vi "Aurora Read Debug Signals (Dual Port).vi"(2 "Debug CLIP Resources":T2={"Hard Error"="Chevelle IO Socket\\uPort0_HardError", "Soft Error"="Chevelle IO Socket\\uPort0_SoftError", "Lane Up"="Chevelle IO Socket\\uPort0_LaneUp", "Channel Up"="Chevelle IO Socket\\uPort0_ChannelUp", "Sys Reset"="Chevelle IO Socket\\uPort0_sys_reset_out"}) -> (4 "Debug Info":T1)   [LabVIEW 2019]
doc: "Reads debug signals from the CLIP.\n\n<B>Input Parameters</B>\n\n<B>Debug CLIP Resources</B> specifies the CLIP Resources used for debug signals.\n\n<B>Debug CLIP Resources.Hard Error</B> specifies the CLIP Resource used to indicate a Hard Error.\n\n<B>Debug CLIP Resources.Soft Error</B> specifies the CLIP Resource used to indicate a Soft Error.\n\n<B>Debug CLIP Resources.Lane Up</B> specifies the CLIP Resource used to indicate whether the Lane is Up.\n\n<B>Debug CLIP Resources.Channel Up</B> specifies the CLIP Resource used to indicate whether the Channel is Up.\n\n<B>Debug CLIP Resources.Sys Reset</B> specifies the CLIP Resource used to indicate if the System is in Reset.\n\n<B>Output Parameters</B>\n\n<B>Debug Info</B> contains debug information read from the CLIP.\n\n<B>Debug Info.Hard Error</B> indicates whether a Hard Error has occurred.\n\n<B>Debug Info.Soft Error</B> indicates whether a Soft Error has occurred.\n\n<B>Debug Info.Lane Up</B> indicates whether the Lane is Up.\n\n<B>Debug Info.Channel Up</B> indicates whether the Channel is Up.\n\n<B>Debug Info.Sys Reset</B> indicates whether the System is in Reset."
uses:
  <vilib>/eio/EIONode/EIONode.xnode
  <vilib>/rvi/eio/common/nirviEmuTemplateMethod_errors.vi
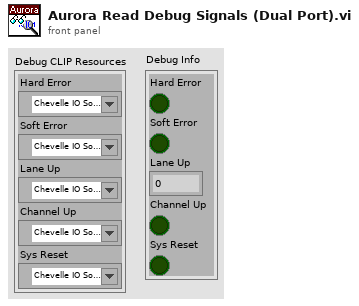
[diagram p1: front panel]
types:
  T1 = cluster{"Hard Error":bool, "Soft Error":bool, "Lane Up":fxp<+,8,8>, "Channel Up":bool, "Sys Reset":bool}
  T2 = cluster{"Hard Error":refnum<k21>, "Soft Error":refnum<k21>, "Lane Up":refnum<k21>, "Channel Up":refnum<k21>, "Sys Reset":refnum<k21>}
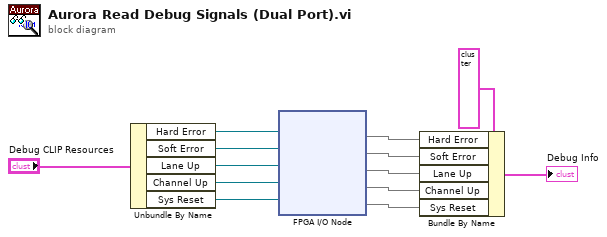
[diagram p0: block diagram]
diagram:
  n1 = Unbundle By Name("Debug CLIP Resources") -> ("Hard Error"=w1:refnum<k21>, "Soft Error"=w12:refnum<k21>, "Lane Up"=w2:refnum<k21>, "Channel Up"=w11:refnum<k21>, "Sys Reset"=w10:refnum<k21>)
  n2 = xnode "FPGA I/O Node"("FPGA I/O In"=w1, "FPGA I/O In"=w12, "FPGA I/O In"=w2, "FPGA I/O In"=w11, "FPGA I/O In"=w10) -> ("I/O Item"=w9, "I/O Item"=w8, "I/O Item"=w3, "I/O Item"=w7, "I/O Item"=w6)  [unwired: 5 out]
  n3 = Bundle By Name(cluster=T1 {"Hard Error"=FALSE, "Soft Error"=FALSE, "Lane Up"=0.0, "Channel Up"=FALSE, "Sys Reset"=FALSE} ("Debug Info 2"), "Hard Error"=w9, "Soft Error"=w8, "Lane Up"=w3, "Channel Up"=w7, "Sys Reset"=w6) -> (→"Debug Info":T1)
